vi "Test SD 1.vi"() -> ()   [LabVIEW 2014]
uses:
  File.lvclass
  LabVIEW Universal Transcriptor SD Card Library.lvlib
panel:
  out "string":string
  out "error out":errorcluster
  in  "Error In":errorcluster
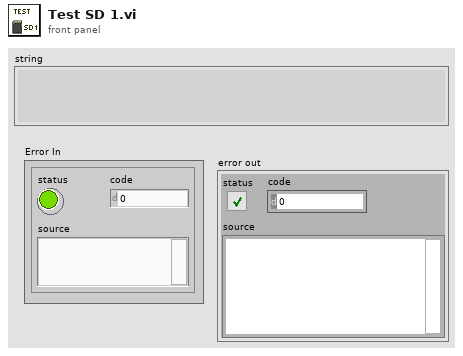
[diagram p1: front panel]
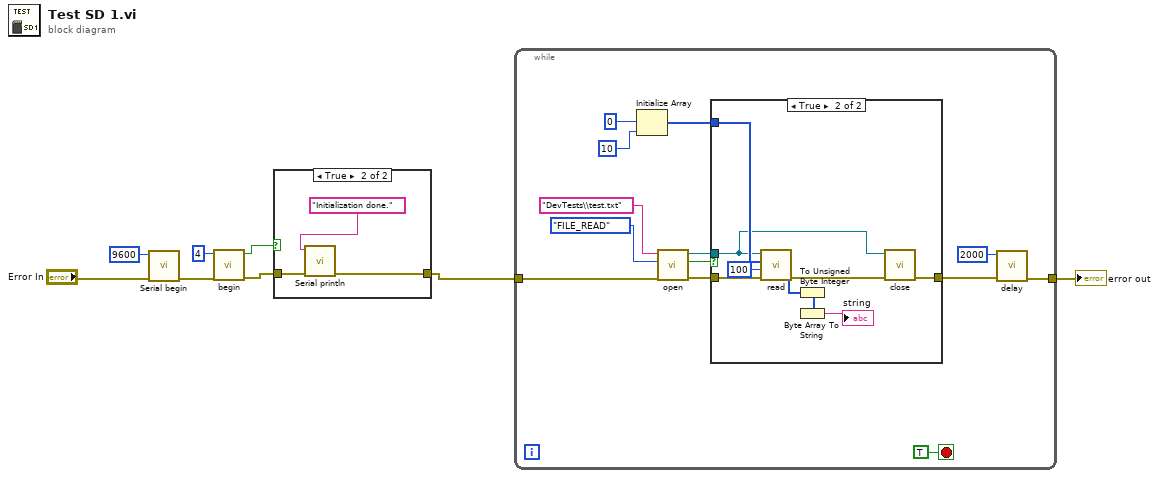
[diagram p0: block diagram]
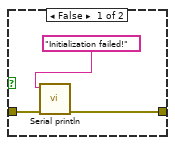
[diagram p3: hidden frame]
diagram:
  n1 = call <vilib>:"Serial begin.vi"("Error In"="Error In", "speed (Bd)"=9600) -> ("Error Out"=w7:errorcluster)  [unwired: 9 in]
  n2 = call "begin.vi"("Error In"=w7, "CS pin (optional)"=u8 4) -> ("Error Out"=w4:errorcluster, "success?"=w3:bool)  [unwired: 8 in]
  n3 = case shown="True" w3 {
    tunnel: w4 -> [w10 w13]
    tunnel: [w9 w12] -> w2
    frame False {
      n4 = call <vilib>:"Serial println.vi"("Error In"=w10, "string in"="Initialization failed!" ("filepath")) -> ("Error Out"=w9:errorcluster)  [unwired: 9 in]
    }
    frame True {
      n5 = call <vilib>:"Serial println.vi"("Error In"=w13, "string in"="Initialization done." ("filepath")) -> ("Error Out"=w12:errorcluster)  [unwired: 9 in]
    }
  }
  n6 = while {
    tunnel: w2 -> [w25]
    tunnel: [w23] -> w1
    stop <- TRUE stop-if-true
    n7 = Initialize Array(i8 0, 10) -> (w16:i8[])
    n8 = call "open.vi"("Error In"=w25, "mode"=enum16{"FILE_READ", "FILE_WRITE"}."FILE_READ", "filepath"="DevTests\\test.txt") -> ("Error Out"=w18:errorcluster, "opened?"=w15:bool, "File out"=w19:refnum<class "File.lvclass">)  [unwired: 6 in]
    n9 = case shown="True" w15 {
      tunnel: w19 -> [_ w33]
      tunnel: w18 -> [w28 w36]
      tunnel: [w28 w37] -> w17
      tunnel: w16 -> [_ w35]
      frame False {
      }
      frame True {
        n10 = call-dynamic "read.vi"("error in (no error)"=w36, "length"=100, "buffer"=w35, "File in"=w33) -> ("error out"=w32:errorcluster, "output buffer"=w31:i8[])  [unwired: 6 in]
        n11 = To Unsigned Byte Integer(number=w31) -> (unsigned 8bit integer=w30:u8[])
        n12 = Byte Array To String(unsigned byte array=w30) -> (string=→"string":string)
        n13 = call-dynamic "close.vi"("error in (no error)"=w32, "File in"=w33) -> ("error out"=w37:errorcluster)  [unwired: 9 in]
      }
    }
    n14 = call <vilib>:"delay.vi"("Error In"=w17, "time (ms)"=2000) -> ("Error Out"=w23:errorcluster)  [unwired: 9 in]
  }
  "error out" <- w1
